vi "CloseAll.vi"(8 "error in (no error)":errorcluster, 11 "sub-systems in":refnum<class "sub-systems.lvclass">) -> (0 "error out":errorcluster, 3 "sub-systems out":refnum<class "sub-systems.lvclass">)   [LabVIEW 2018, in "sub-systems.lvclass"]
uses:
  sub-systems.lvclass
  sub-systems.lvclass/sub-systems.ctl
  VSMx2/VXMx2.lvclass
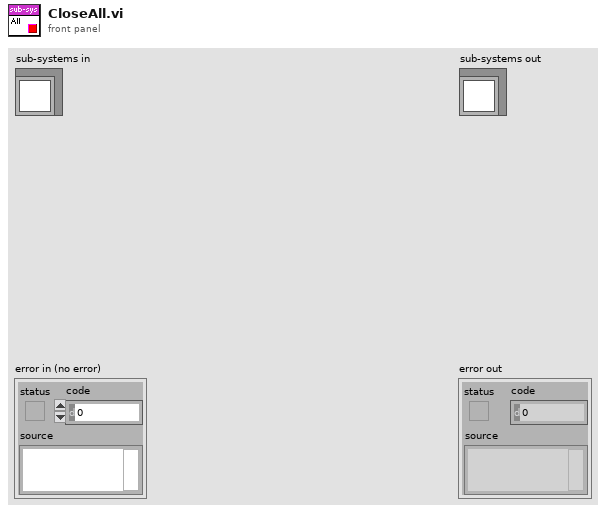
[diagram p1: front panel]
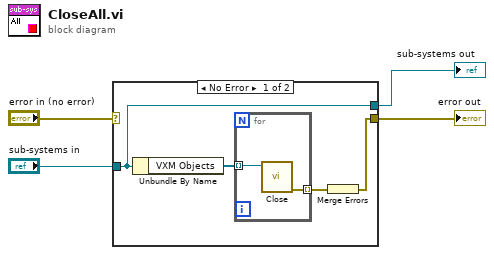
[diagram p0: block diagram]
diagram:
  n1 = case shown="No Error" "error in (no error)" {
    selector: "error in (no error)" -> [_ w12]
    tunnel: [w5 w12] -> w3
    tunnel: [w8 w11] -> w1
    tunnel: "sub-systems in" -> [w8 w11]
    frame No Error {
      n2 = Unbundle By Name(w8) -> ("VXM Objects"=w7:refnum<class "VXMx2.lvclass">[])
      n3 = for {
        tunnel: w7 -> [w10] mode=indexing
        tunnel: [w9] -> w6 mode=indexing
        n4 = call "Close.vi"("VXMx2 in"=w10) -> ("error out"=w9:errorcluster)  [unwired: 9 in, 1 out]
      }
      n5 = Merge Errors(w6) -> (w5:errorcluster)
    }
    frame Error {
    }
  }
  "error out" <- w3
  "sub-systems out" <- w1
